vi "Indexer PID.vi"(11 "Time Delay Milli":dbl) -> ()   [LabVIEW 2011]
uses:
  Actual RPM Global.vi
  PID Set Points.vi
  <vilib>/addons/control/pid/pid.llb/PID (DBL).vi
  <vilib>/addons/control/pid/NI_PID_pid.lvlib
panel:
  out "Distance":dbl
  in  "Graph time interval  in seconds":dbl
  out "Indexer RPM":cluster{dbl, dbl, dbl[]}(graph)
  out "RPM Error 2":dbl
  out "Encoder Speed":dbl
  in  "D 2":dbl
  in  "I 2":dbl
  in  "P 2":dbl=0.01 step=0.001
  out "Encoder Set Speed 2":dbl
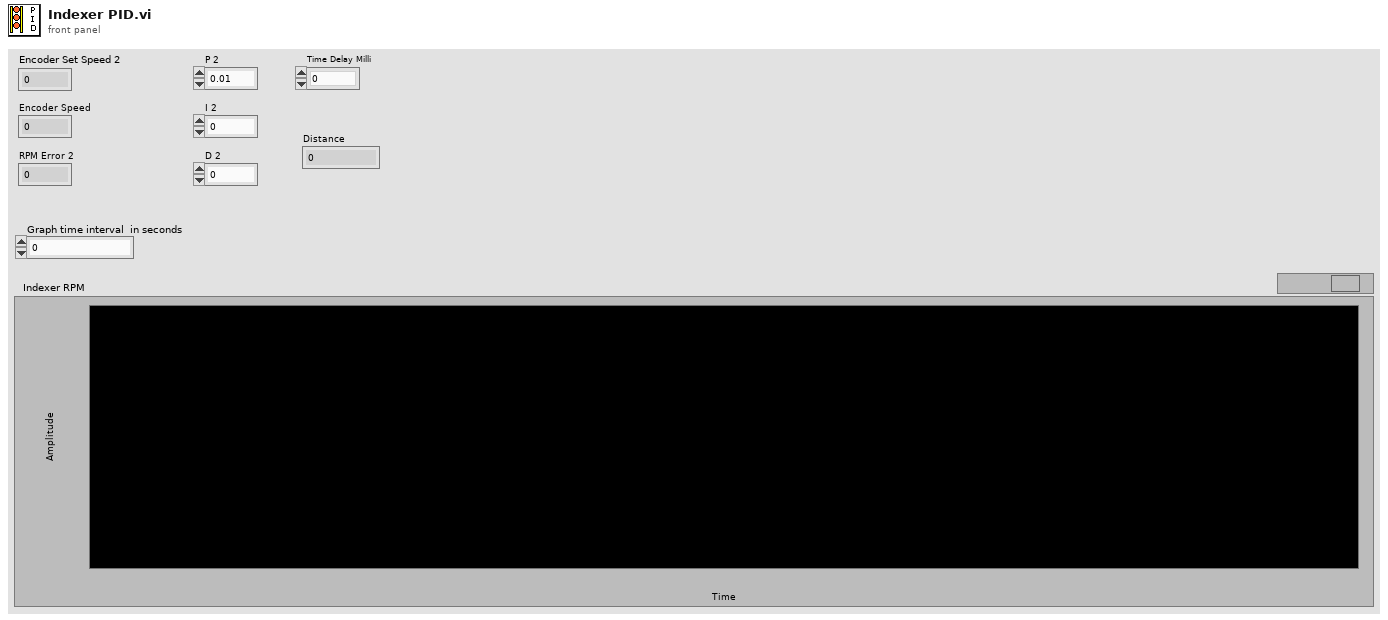
[diagram p1: front panel]
types:
  T1 = typedef "WPI_EncoderDevRef.ctl" = cluster{"DevStatus":errorcluster, "EncoderIndex":T2, "CounterIndex":T3, "DistancePerCount":dbl, "Decoding Type":T4}
  T2 = typedef "FPGA_EncoderIdx.ctl" = enum8{"Enc 0", "Enc 1", "Enc 2", "Enc 3", "Invalid"}
  T3 = typedef "FPGA_CounterCtrSystemIndex.ctl" = enum8{"Ctr 0", "Ctr 1", "Ctr 2", "Ctr 3", "Ctr 4", "Ctr 5", "Ctr 6", "Ctr 7", "Invalid"}
  T4 = typedef "WPI_EncoderType.ctl" = enum16{"1x", "2x", "4x"}
  T5 = typedef "WPI_MotorControlDeviceRef.ctl" = cluster{"DeviceStatus":errorcluster, "Type":enum16{"PWM", "CAN"}, "PWM":cluster{"Digital Module":T6, "PWM Channel":T7, "DeadBand":T8}, "CAN":cluster{"Device Number":u8, "Control Mode":T9, "Semaphore":T10, "Max Vout":dbl}, "Invert":bool, "TransformRef":T11, "InvTransformRef":T11}
  T6 = typedef "FPGA_TypedefDigitalModule.ctl" = enum16{"Digital Module 1", "Digital Module 2"}
  T7 = typedef "FPGA_DIOPWMChannel.ctl" = enum8{"PWM 1", "PWM 2", "PWM 3", "PWM 4", "PWM 5", "PWM 6", "PWM 7", "PWM 8", "PWM 9", "PWM 10", "Invalid"}
  T8 = typedef "WPI_PWMDeadband.ctl" = cluster{"Name":string, "maxPositivePwm":i32, "minPositivePwm":i32, "centerPwm":i32, "maxNegativePwm":i32, "minNegativePwm":i32, "angularRange":u16}
  T9 = typedef "WPI_CANJaguar_ControlMode.ctl" = enum8{"Percent VBus", "Current", "Speed", "Position", "Voltage"}
  T10 = typedef "Semaphore RefNum" = refnum<k1>
  T11 = typedef "WPI_PWMTransform_ConPane.ctl" = refnum<vi>
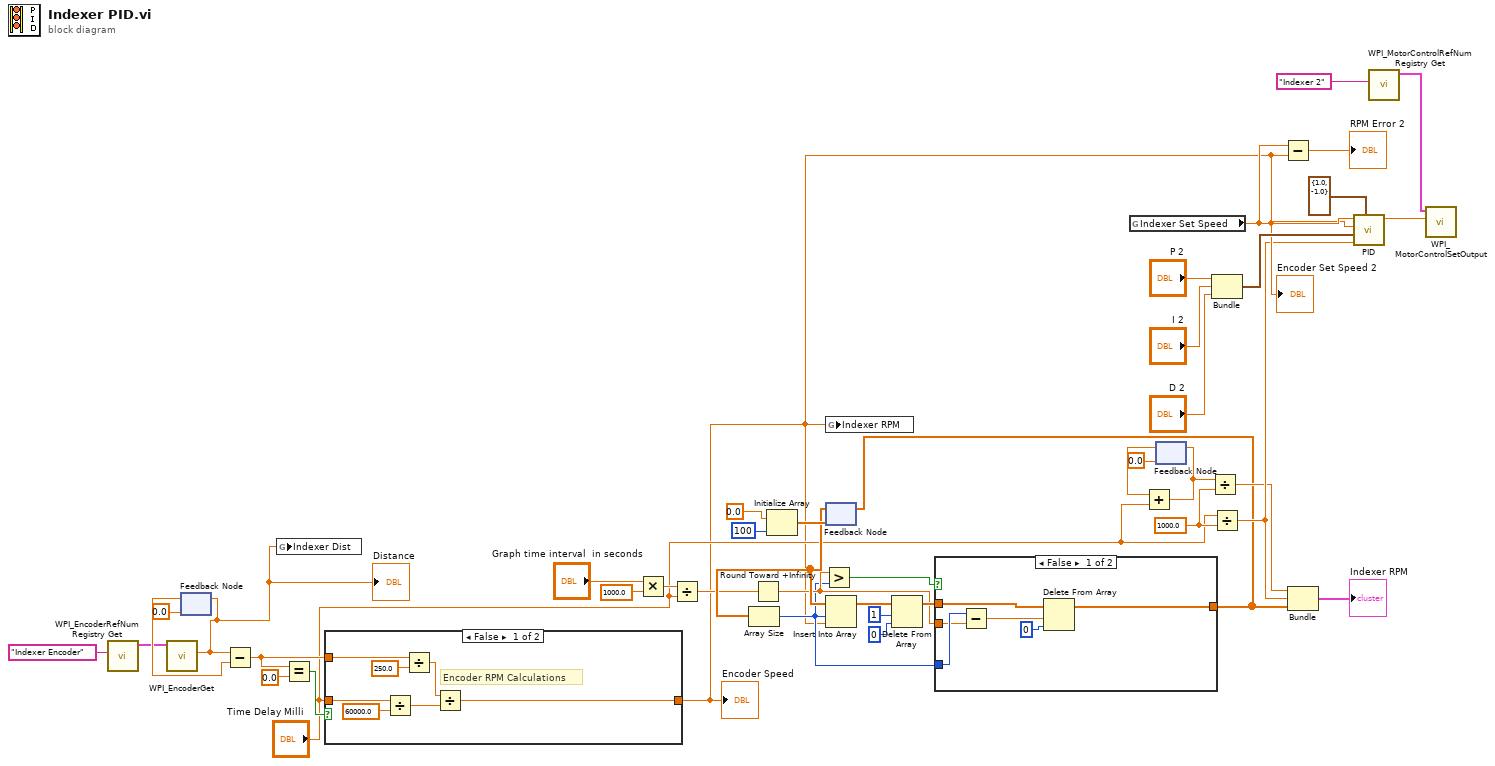
[diagram p0: block diagram]
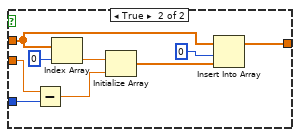
[diagram p2: hidden frame]
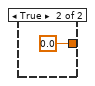
[diagram p3: hidden frame]
diagram:
  w16 = 1000.0 ("y")
  n1 = call <vilib>:"WPI_EncoderRefNum Registry Get.vi"("refnum name"="Indexer Encoder") -> ("EncoderDevRef"=w25:T1)  [unwired: 9 in, 1 out]
  n2 = call <vilib>:"WPI_EncoderGet.vi"("EncoderDevRef"=w25) -> ("Distance"=w1:dbl)  [unwired: 5 in, 5 out]
  "Distance" <- w1
  n3 = feedback #1(0.0) -> (w32:dbl)
  n4 = feedback-in #1(w1) -> ()
  n5 = Subtract(x=w1, y=w32) -> (x-y=w27:dbl)
  n6 = global write "Actual RPM Global.vi" "Indexer Dist"(w1) -> ()
  n7 = Equal?(x=w27, y=0.0) -> (x = y?=w28:bool)
  n8 = case shown="False" w28 {
    tunnel: [w49 0.0] -> w3
    tunnel: w27 -> [w48 _]
    tunnel: "Time Delay Milli" -> [w46 _]
    frame False {
      # "Encoder RPM Calculations"
      n9 = Divide(x=w46, y=60000.0) -> (x/y=w44:dbl)
      n10 = Divide(x=w48, y=250.0) -> (x/y=w47:dbl)
      n11 = Divide(x=w47, y=w44) -> (x/y=w49:dbl)
    }
    frame True {
    }
  }
  "Encoder Speed" <- w3
  n12 = Multiply(x="Graph time interval  in seconds", y=1000.0) -> (x*y=w11:dbl)
  n13 = Divide(x=w11, y="Time Delay Milli") -> (x/y=w9:dbl)
  n14 = Round Toward +Infinity(x=w9) -> (ceil(x): smallest int >= x=w6:dbl)
  n15 = Initialize Array(0.0 ("element"), 100 ("dimension size")) -> (w34:dbl[])
  n16 = global write "Actual RPM Global.vi" "Indexer RPM"(w3) -> ()
  n17 = feedback #2(w34) -> (w22:dbl[])
  n18 = Array Size(array=w22) -> (size(s)=w5:i32)
  n19 = Greater?(x=w6, y=w5) -> (0:w8:bool)
  n20 = Insert Into Array(array=w22, index=w5, new element=w3) -> (w21:dbl[])
  n21 = Delete From Array(array=w21, length=1, index=0) -> (array with subset deleted=w7:dbl[])  [unwired: 1 out]
  n22 = case shown="False" w8 {
    tunnel: w7 -> [w53 w65]
    tunnel: w6 -> [w55 w63]
    tunnel: w5 -> [w56 w62]
    tunnel: [w52 w58] -> w4
    frame False {
      n23 = Subtract(x=w56, y=w55) -> (x-y=w54:dbl)
      n24 = Delete From Array(array=w53, length=w54, index=0) -> (array with subset deleted=w52:dbl[])  [unwired: 1 out]
    }
    frame True {
      n25 = Subtract(x=w63, y=w62) -> (x-y=w61:dbl)
      n26 = Index Array(array=w65, index=0) -> (element=w66:dbl)
      n27 = Initialize Array(w66, w61) -> (w60:dbl[])
      n28 = Insert Into Array(array=w65, index=0, new element=w60) -> (w58:dbl[])
    }
  }
  n29 = feedback-in #2(w4) -> ()
  n30 = global read "PID Set Points.vi" "Indexer Set Speed"() -> (w35:dbl)
  "Encoder Set Speed 2" <- w35
  n31 = feedback #3(0.0) -> (w17:dbl)
  n32 = Add(x=w17, y="Time Delay Milli") -> (x+y=w14:dbl)
  n33 = feedback-in #3(w14) -> ()
  n34 = Divide(x=w14, y=w16) -> (x/y=w15:dbl)
  n35 = Bundle("P 2"="P 2", "I 2"="I 2", "D 2"="D 2") -> (w39:cluster{"P 2":dbl, "I 2":dbl, "D 2":dbl})  [unwired: 1 in]
  n36 = Divide(x="Time Delay Milli", y=w16) -> (x/y=w23:dbl)
  n37 = Subtract(x=w35, y=w3) -> (x-y=→"RPM Error 2":dbl)
  n38 = Bundle(w15, w23, w4) -> (→"Indexer RPM":cluster{dbl, dbl, dbl[]})  [unwired: 1 in]
  n39 = call-poly <vilib>:"PID.vi"("output range"=cluster{"output high":dbl, "output low":dbl} {"output high"=1.0, "output low"=-1.0}, "dt (s)"=w23, "PID gains"=w39, "process variable"=w3, "setpoint"=w35) -> ("output"=w2:dbl)  [unwired: 5 in, 1 out]
  n40 = call <vilib>:"WPI_MotorControlRefNum Registry Get.vi"("refnum name"="Indexer 2") -> ("MotorControlDevRef"=w36:T5)  [unwired: 9 in, 1 out]
  n41 = call <vilib>:"WPI_MotorControlSetOutput.vi"("Output"=w2, "MotorControlDevRef"=w36) -> ()  [unwired: 8 in, 2 out]
